vi "test_CCDAcquisitionSequence.vi"(7 "Test should pass":bool=TRUE, 8 "error in":errorcluster, 9 "tear down connection":bool=TRUE, 10 "set-up a connection":bool=TRUE, 11 "device selection":enum16{"monochromator", "CCD", "SCD"}(ring)=enum."CCD") -> (0 "error out":errorcluster)   [LabVIEW 2023]
uses:
  <vilib>/addons/_JKI Toolkits/Caraya/classes/Test/Test.lvclass
  <vilib>/addons/_JKI Toolkits/Caraya/classes/Assert/Assert.lvclass
  Source/Classes/CCD/CCD.lvclass
  Source/Classes/SCD/SCD.lvclass
  Source/Classes/Mono/Monochromator.lvclass
  <vilib>/addons/_JKI Toolkits/Caraya/classes/Assert/Assert Not Error.vi
  <vilib>/addons/_JKI Toolkits/Caraya/classes/Assert/Assert Equal Value and Type_Variant.vi
panel:
  # "Connector Pane"
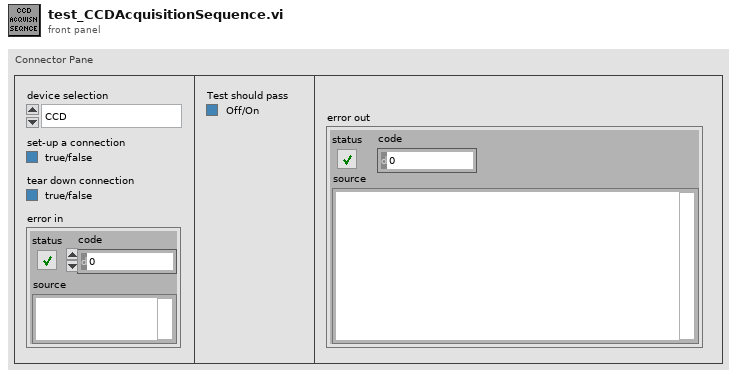
[diagram p1: front panel]
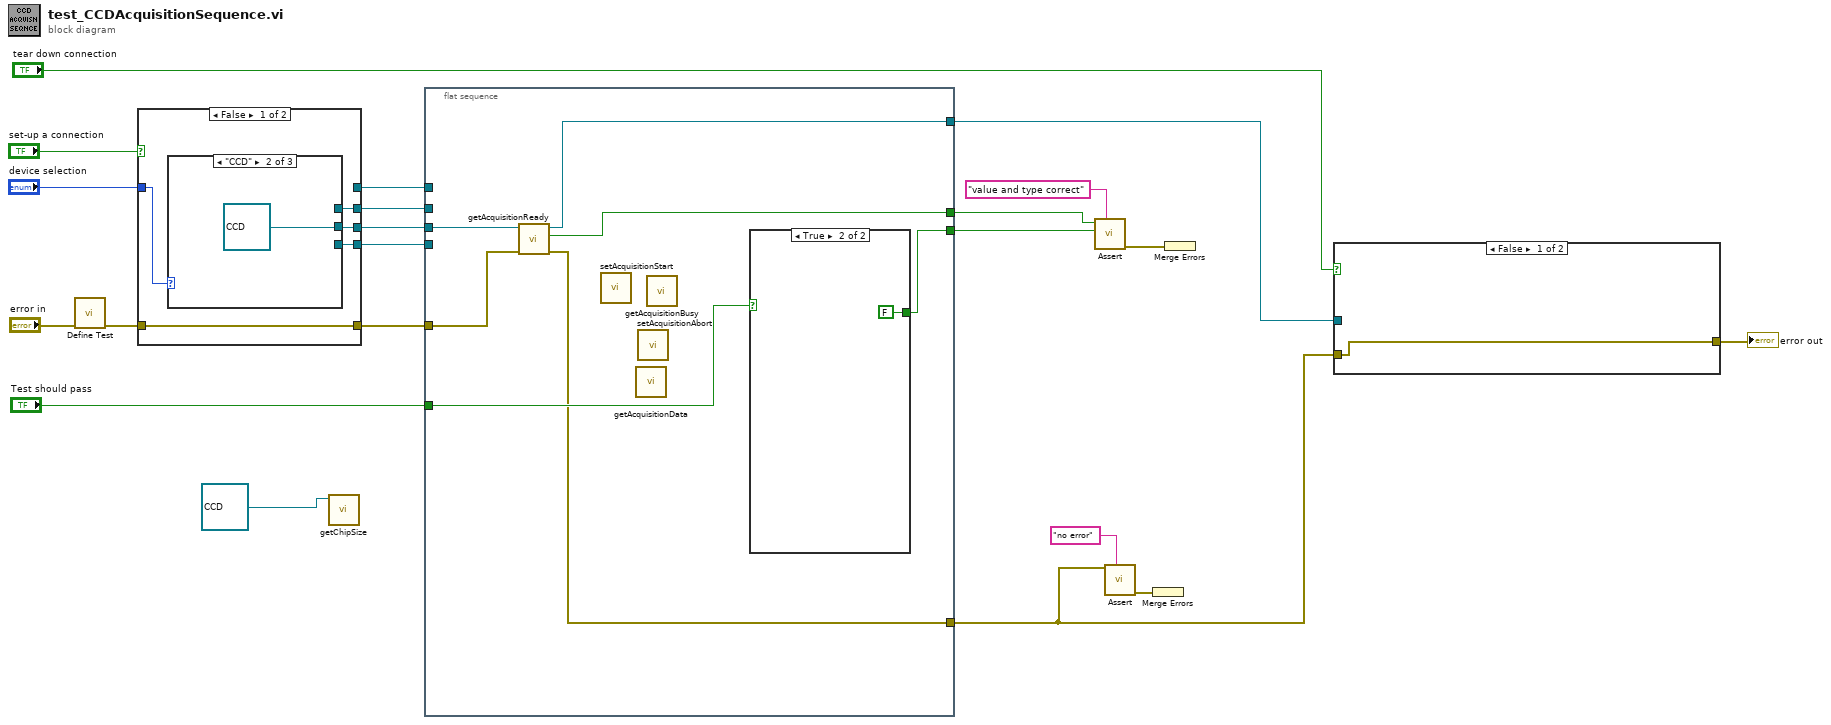
[diagram p0: block diagram]
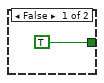
[diagram p2: hidden frame]
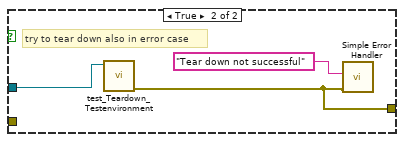
[diagram p3: hidden frame]
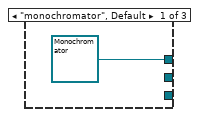
[diagram p4: hidden frame]
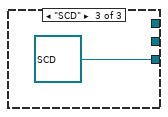
[diagram p5: hidden frame]
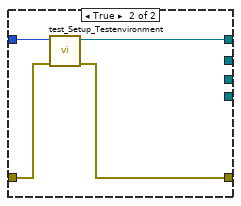
[diagram p6: hidden frame]
diagram:
  n1 = call <vilib>:"Define Test.vi"("error in (no error)"="error in") -> ("error out"=w14:errorcluster)  [unwired: 9 in, 1 out]
  n2 = case shown="False" "set-up a connection" {
    tunnel: w14 -> [w26 w33]
    tunnel: [w26 w32] -> w16
    tunnel: "device selection" -> [w25 w31]
    tunnel: [_ w30] -> w13
    tunnel: [w24 _] -> w12
    tunnel: [w23 _] -> w11
    tunnel: [w22 _] -> w10
    frame False {
      n3 = case shown="\"CCD\"" w25 {
        tunnel: [refnum<class "Monochromator.lvclass"> refnum ("Monochromator.lvclass") _ _] -> w24
        tunnel: [_ refnum<class "CCD.lvclass"> refnum ("CCD in") _] -> w23
        tunnel: [_ _ refnum<class "SCD.lvclass"> refnum ("SCD.lvclass")] -> w22
        frame "monochromator", Default {
        }
        frame "CCD" {
        }
        frame "SCD" {
        }
      }
    }
    frame True {
      n4 = call "test_Setup_Testenvironment.vi"("error in"=w33, "device selection"=w31) -> ("error out"=w32:errorcluster, "GenericDevice.lvclass"=w30:refnum<class "GenericDevice.lvclass">)  [unwired: 7 in, 1 out]
    }
  }
  n5 = call-dynamic "getChipSize.vi"("CCD in"=refnum<class "CCD.lvclass"> refnum) -> ()  [unwired: 7 in, 4 out]
  n6 = flat-sequence {
    tunnel: [w35] -> w18
    tunnel: w16 -> [w38]
    tunnel: w13 -> [_]
    tunnel: w12 -> [_]
    tunnel: w11 -> [w39]
    tunnel: w10 -> [_]
    tunnel: [w37] -> w5
    tunnel: "Test should pass" -> [w40]
    tunnel: [w36] -> w4
    tunnel: [w34] -> w1
    frame #0 {
      n7 = call "getAcquisitionReady.vi"("error in (no error)"=w38, "CCD in"=w39) -> ("error out"=w37:errorcluster, "ready"=w35:bool, "CCD out"=w36:refnum<class "CCD.lvclass">)  [unwired: 7 in]
      n8 = call "setAcquisitionStart.vi"() -> ()  [unwired: 8 in, 4 out]
      n9 = call "getAcquisitionData.vi"() -> ()  [unwired: 10 in, 2 out]
      n10 = call "setAcquisitionAbort.vi"() -> ()  [unwired: 8 in, 4 out]
      n11 = call "getAcquisitionBusy.vi"() -> ()  [unwired: 9 in, 3 out]
      n12 = case shown="True" w40 {
        tunnel: [TRUE FALSE] -> w34
        frame False {
        }
        frame True {
        }
      }
    }
  }
  n13 = call-poly <vilib>:"Assert.vi"("Label"="value and type correct" ("Label (VI Title)"), "Y"=w1, "X"=w18) -> ("error out"=w19:errorcluster)  [unwired: 7 in, 1 out]
  n14 = call-poly <vilib>:"Assert.vi"("Label"="no error" ("Label (VI Title)"), "Not Error?"=w5) -> ("error out"=w7:errorcluster)  [unwired: 8 in, 1 out]
  n15 = Merge Errors(w7) -> ()  [unwired: 1 out]
  n16 = Merge Errors(w19) -> ()  [unwired: 1 out]
  n17 = case shown="False" "tear down connection" {
    tunnel: w4 -> [_ w45]
    tunnel: [w43 w44] -> w3
    tunnel: w5 -> [w43 _]
    frame False {
    }
    frame True {
      # "try to tear down also in error case"
      n18 = call "test_Teardown_Testenvironment.vi"("GenericDevice.lvclass"=w45) -> ("error out"=w44:errorcluster)  [unwired: 9 in, 1 out]
      n19 = call <vilib>:"Simple Error Handler.vi"("error source (\" \")"="Tear down not successful" ("error source (\" \")"), "error in (no error)"=w44) -> ()  [unwired: 3 in, 5 out]
    }
  }
  "error out" <- w3
